vi "LV-Data-V3.vi"() -> ()   [LabVIEW 2025]
uses:
  <vilib>/DAQmx/read.llb/DAQmx Read (Analog DBL 1Chan 1Samp).vi
  <vilib>/DAQmx/create/channels.llb/DAQmx Create Channel (AI-Voltage-Basic).vi
  <vilib>/DAQmx/miscellaneous.llb/DAQmx Fill In Error Info.vi
panel:
  out "time (ms)":u32
  in  "Filename":path
  in  "Enable":bool=TRUE
  in  "sample frequency (Hz)":u32=20
  out "Waveform Chart":dbl(graph)
  in  "stop/save file":bool
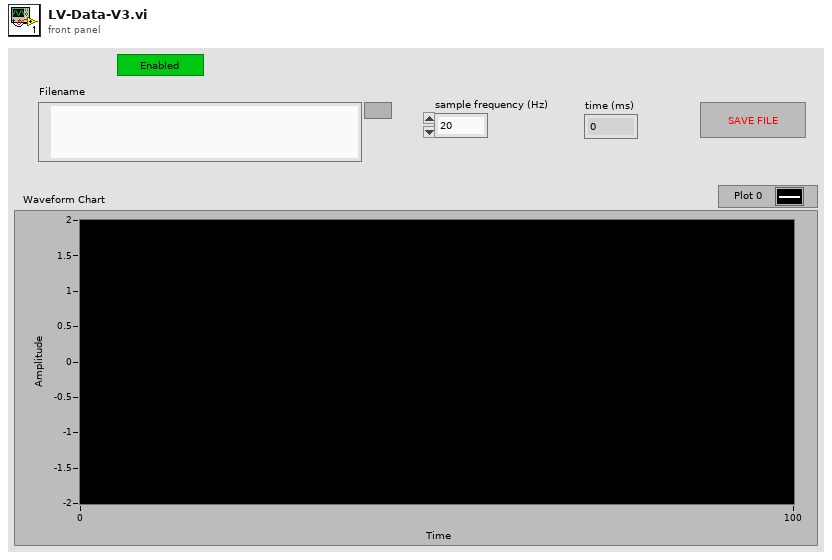
[diagram p1: front panel]
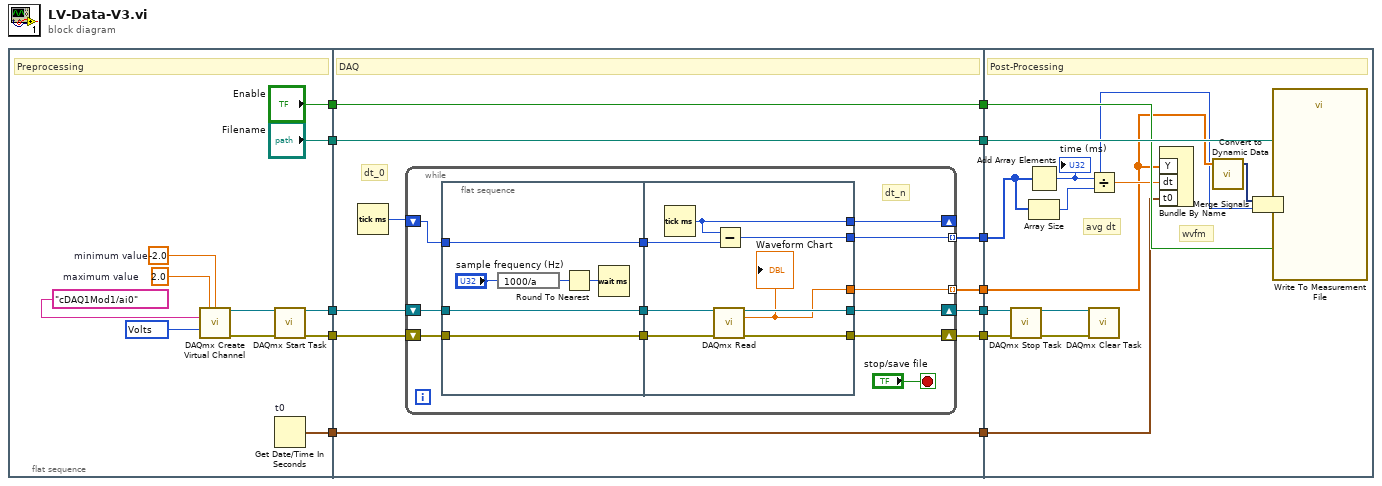
[diagram p0: block diagram]
diagram:
  n1 = flat-sequence {
    tunnel: [w17] -> w10
    tunnel: [w16] -> w9
    tunnel: ["Filename"] -> w7
    tunnel: ["Enable"] -> w5
    tunnel: [w13] -> w2
    tunnel: [w33] -> w12
    tunnel: [w32] -> w11
    tunnel: w10 -> [w31]
    tunnel: w9 -> [w30]
    tunnel: [w29] -> w8
    tunnel: w7 -> [w29]
    tunnel: [w28] -> w6
    tunnel: w5 -> [w28]
    tunnel: [w26] -> w4
    tunnel: [w25] -> w3
    tunnel: w2 -> [w25]
    tunnel: [w24] -> w1
    tunnel: w12 -> [w71]
    tunnel: w11 -> [w70]
    tunnel: w8 -> [w69]
    tunnel: w6 -> [w68]
    tunnel: w4 -> [w67]
    tunnel: w3 -> [w64]
    tunnel: w1 -> [w63]
    frame #0 {
      w20 = -2.0  # minimum value
      w21 = 2.0  # maximum value
      w18 = 10348 items=["Volts"=10348, "From Custom Scale"=10065] ("units")
      # "Preprocessing"
      n2 = call-poly <vilib>:"DAQmx Create Virtual Channel.vi"("maximum value"=w21, "minimum value"=w20, "physical channels"=tag "cDAQ1Mod1/ai0", "units"=w18) -> ("task out"=w22:refnum<k21>, "error out"=w23:errorcluster)  [unwired: 10 in]
      n3 = call <vilib>:"DAQmx Start Task.vi"("task/channels in"=w22, "error in"=w23) -> ("task out"=w17:refnum<k21>, "error out"=w16:errorcluster)  [unwired: 12 in]
      n4 = Get Date/Time In Seconds "t0"() -> (seconds since 1Jan1904=w13:timestamp)
    }
    frame #1 {
      # "dt_0"
      # "DAQ"
      n5 = Tick Count (ms)() -> (millisecond timer value=w27:u32)
      n6 = while {
        shift-right: [w43] -> w33
        shift-left: w31 -> [w45]
        shift-right: [w42] -> w32
        shift-left: w30 -> [w44]
        shift-right: [w36] -> _
        shift-left: w27 -> [w37]
        tunnel: [w35] -> w26 mode=indexing
        tunnel: [w34] -> w24 mode=indexing
        stop <- "stop/save file" stop-if-true
        # "dt_n"
        n7 = flat-sequence {
          tunnel: w44 -> [w50]
          tunnel: w45 -> [w51]
          tunnel: [w51] -> w40
          tunnel: [w50] -> w39
          tunnel: [w49] -> w38
          tunnel: w37 -> [w49]
          tunnel: [w57] -> w43
          tunnel: [w56] -> w42
          tunnel: w40 -> [w59]
          tunnel: w39 -> [w58]
          tunnel: w38 -> [w55]
          tunnel: [w54] -> w36
          tunnel: [w53] -> w35
          tunnel: [w52] -> w34
          frame #0 {
            n8 = expression code="1000/a"("sample frequency (Hz)") -> (w47:u32)
            n9 = Round To Nearest(number=w47) -> (nearest integer value=w46:u32)
            n10 = Wait (ms)(milliseconds to wait=w46) -> ()  [unwired: 1 out]
          }
          frame #1 {
            n11 = Tick Count (ms)() -> (millisecond timer value=w54:u32)
            n12 = call-poly <vilib>:"DAQmx Read.vi"("task/channels in"=w59, "error in"=w58) -> ("task out"=w57:refnum<k21>, "data"=w52:dbl, "error out"=w56:errorcluster)  [unwired: 11 in]
            "Waveform Chart" <- w52
            n13 = Subtract(x=w54, y=w55) -> (x-y=w53:u32)
          }
        }
      }
    }
    frame #2 {
      # "wvfm"
      # "avg dt"
      # "Post-Processing"
      n14 = call <vilib>:"DAQmx Stop Task.vi"("task/channels in"=w71, "error in"=w70) -> ("task out"=w72:refnum<k21>, "error out"=w73:errorcluster)  [unwired: 12 in]
      n15 = Add Array Elements(numeric array=w67) -> (sum=w60:u32)
      "time (ms)" <- w60
      n16 = Array Size(array=w67) -> (size(s)=w66:i32)
      n17 = Divide(x=w60, y=w66) -> (x/y=w65:dbl)
      n18 = call <vilib>:"DAQmx Clear Task.vi"("task in"=w72, "error in"=w73) -> ()  [unwired: 13 in, 1 out]
      n19 = Bundle By Name("Y"=w63, "dt"=w65, "t0"=w64) -> ()  [unwired: 1 in, 1 out]
      n20 = call "Convert to Dynamic Data"("Array"=w63) -> ("Dynamic Data Type"=w62:dynamicdata)  [unwired: 3 in]
      n21 = Merge Signals(w62, w60) -> (w61:dynamicdata)
      n22 = call "Write To Measurement File"("Signals"=w61, "Enable"=w68, "Filename"=w69) -> ()  [unwired: 14 in, 3 out]
    }
  }
